vi "Initialize.vi"(8 "error in (no error)":errorcluster {"code" format="%.0x"}, 9 "reset device (Off)":bool, 10 "id query (Off)":bool, 11 "resource name":refnum<k15> caption="resource string") -> (0 "error out":errorcluster {"code" format="%.0x"}, 3 "instrument handle out":refnum<k15>)   [LabVIEW 2021, in "Keysight XSAnVMA.lvlib"]
doc: "Opens the I/O session to the instrument. Driver methods and properties that access the instrument are only accessible after Initialize is called. Initialize optionally performs a Reset and queries the instrument to validate the instrument model."
uses:
  <instrlib>/Keysight XSAnVMA/Keysight XSAnVMA.lvlib
panel:
  # "© Keysight Technologies 2018-2019"
  # "© 2000-2008 National Instruments.  All Rights Reserved."
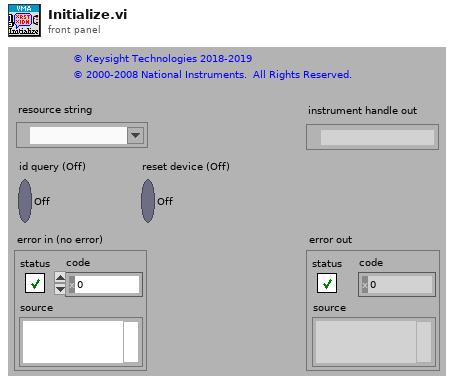
[diagram p1: front panel]
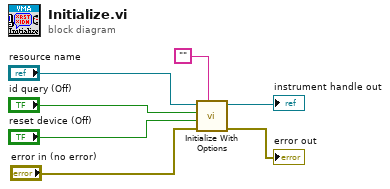
[diagram p0: block diagram]
diagram:
  n1 = call "Initialize With Options.vi"("option string"="", "error in (no error)"="error in (no error)", "reset device (Off)"="reset device (Off)", "id query (Off)"="id query (Off)", "resource string"="resource name") -> ("error out"=→"error out":errorcluster, "instrument handle out"=→"instrument handle out":refnum<k15>)  [unwired: 5 in]
